vi "Get Addresses for Activation.vi"(8 "error in (no error)":errorcluster, 10 "config file refnum in":T1, 11 "IED in":refnum<class "IED.lvclass">) -> (0 "error out":errorcluster, 2 "config file refnum out":T1, 3 "IED out":refnum<class "IED.lvclass">)   [LabVIEW 2015, in "IED Actor.lvlib" / "IED.lvclass"]
uses:
  IED.lvclass
  <vilib>/Utility/config.llb/Config Data RefNum.ctl
  IED.lvclass/IED.ctl
  <vilib>/Utility/config.llb/Read Key (U32).vi
  <vilib>/Modbus/master/Modbus Master.lvclass
  <vilib>/Utility/config.llb/NI_LVConfig.lvlib
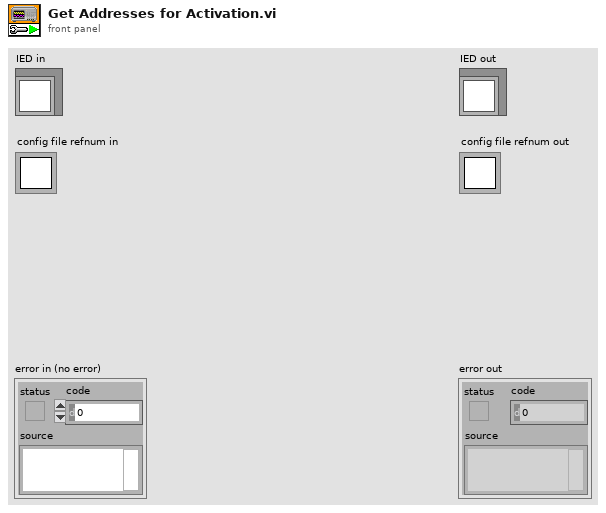
[diagram p1: front panel]
types:
  T1 = typedef "NI_LVConfig.lvlib/Config Data RefNum.ctl" = refnum<k1>
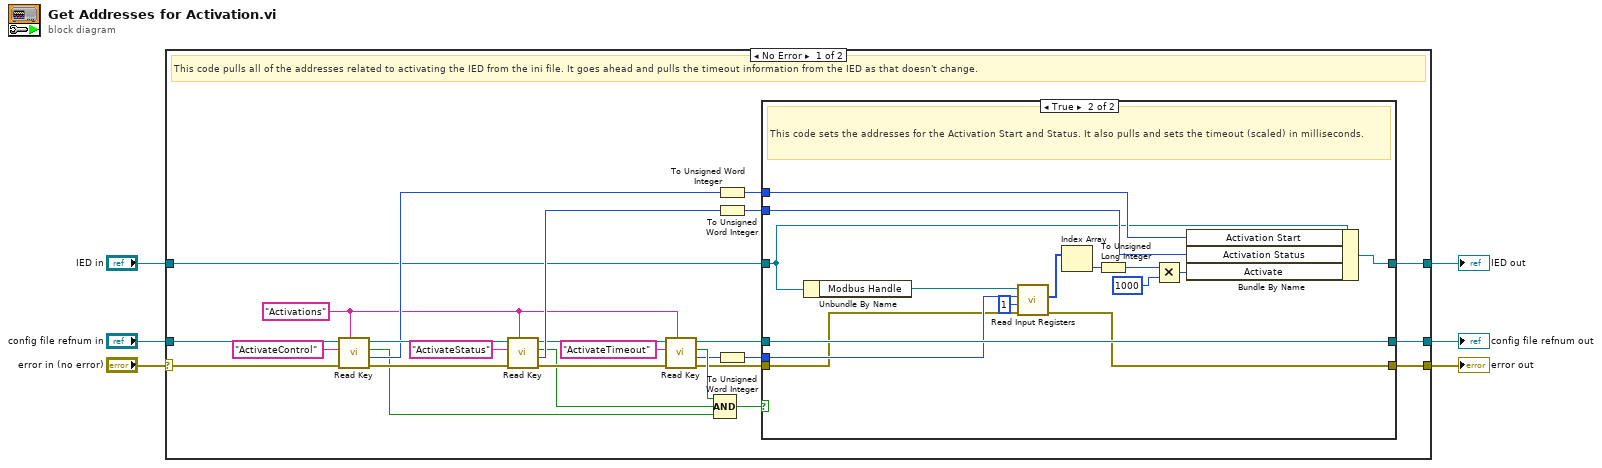
[diagram p0: block diagram]
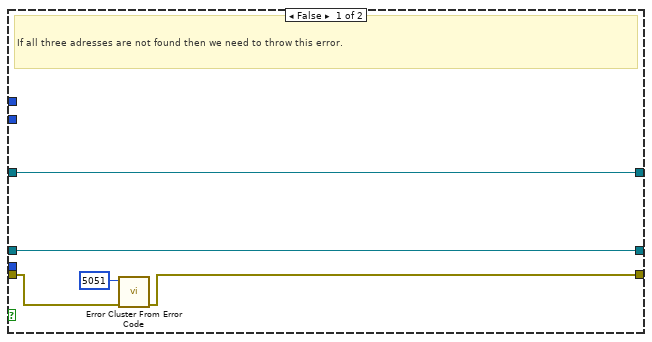
[diagram p2: hidden frame]
diagram:
  n1 = case shown="No Error" "error in (no error)" {
    selector: "error in (no error)" -> [w31 w55]
    tunnel: [w11 w55] -> w5
    tunnel: [w10 w54] -> w3
    tunnel: "IED in" -> [w12 w54]
    tunnel: "config file refnum in" -> [w32 w53]
    tunnel: [w9 w53] -> w1
    frame No Error {
      w21 = "Activations" ("section")
      # "This code pulls all of the addresses related to activating the IED from the ini file. It goes ahead and pulls the timeout information from the IED as that doesn't change."
      n2 = call-poly <vilib>:"Read Key.vi"("section"=w21, "error in (no error)"=w31, "key"="ActivateControl", "refnum"=w32) -> ("error out"=w29:errorcluster, "value"=w26:u32, "found?"=w18:bool, "refnum out"=w28:T1)  [unwired: 4 in]
      n3 = call-poly <vilib>:"Read Key.vi"("section"=w21, "error in (no error)"=w29, "key"="ActivateStatus", "refnum"=w28) -> ("error out"=w23:errorcluster, "value"=w25:u32, "found?"=w19:bool, "refnum out"=w24:T1)  [unwired: 4 in]
      n4 = call-poly <vilib>:"Read Key.vi"("section"=w21, "error in (no error)"=w23, "key"="ActivateTimeout", "refnum"=w24) -> ("error out"=w15:errorcluster, "value"=w7:u32, "found?"=w20:bool, "refnum out"=w16:T1)  [unwired: 4 in]
      n5 = Compound Arithmetic op=AND(w20, w19, w18) -> (w17:bool)
      n6 = To Unsigned Word Integer(number=w26) -> (unsigned 16bit integer=w14:u16)
      n7 = To Unsigned Word Integer(number=w25) -> (unsigned 16bit integer=w13:u16)
      n8 = To Unsigned Word Integer(number=w7) -> (unsigned 16bit integer=w8:u16)
      n9 = case shown="True" w17 {
        tunnel: w16 -> [w33 w49]
        tunnel: w15 -> [w37 w39]
        tunnel: w8 -> [_ w48]
        tunnel: w14 -> [_ w52]
        tunnel: w13 -> [_ w51]
        tunnel: w12 -> [w34 w44]
        tunnel: [w35 w40] -> w11
        tunnel: [w34 w50] -> w10
        tunnel: [w33 w49] -> w9
        frame False {
          # "If all three adresses are not found then we need to throw this error."
          n10 = call <vilib>:"Error Cluster From Error Code.vi"("error in (no error)"=w37, "error code (0)"=5051) -> ("error out"=w35:errorcluster)  [unwired: 7 in]
        }
        frame True {
          # "This code sets the addresses for the Activation Start and Status. It also pulls and sets the timeout (scaled) in milliseconds."
          n11 = Unbundle By Name(w44) -> ("Modbus Handle"=w38:refnum<class "Modbus Master.lvclass">)
          n12 = call-dynamic "Read Input Registers.vi"("error in (no error)"=w39, "number of input registers"=u16 1, "starting address"=w48, "Modbus master in"=w38) -> ("error out"=w40:errorcluster, "register values"=w46:u16[])  [unwired: 5 in, 1 out]
          n13 = Index Array(array=w46) -> (element=w47:u16)  [unwired: 1 in]
          n14 = To Unsigned Long Integer(number=w47) -> (unsigned 32bit integer=w42:u32)
          n15 = Multiply(x=w42, y=u32 1000) -> (x*y=w43:u32)
          n16 = Bundle By Name(cluster=w44, "Activation Start"=w52, "Activation Status"=w51, "Activate"=w43) -> (w50:refnum<class "IED.lvclass">)
        }
      }
    }
    frame Error {
    }
  }
  "error out" <- w5
  "IED out" <- w3
  "config file refnum out" <- w1
